vi "RTSequence.Pause.vi"(11 "StimulusProfileReference":refnum<k24>) -> (3 "error out":errorcluster)   [LabVIEW 2013, in "RTSequenceVIs.lvlib"]
uses:
  RTSequenceVIs.lvlib
  NationalInstruments.VeriStand.ClientAPI
  NationalInstruments.VeriStand
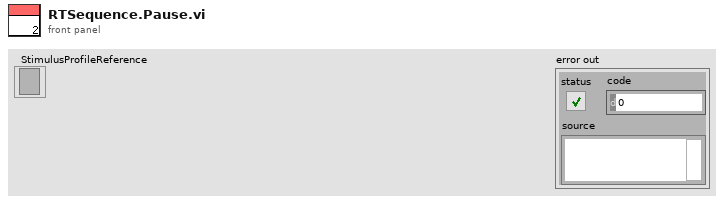
[diagram p1: front panel]
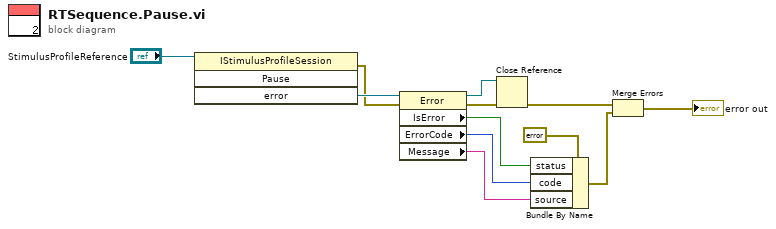
[diagram p0: block diagram]
diagram:
  n1 = invoke class="IStimulusProfileSession" method="Pause"(reference="StimulusProfileReference") -> (error out=w11:errorcluster, "error"=w12:refnum<k24>)  [unwired: 3 in, 2 out]
  n2 = property class="Error"(reference=w12, error in=w11) -> (reference out=w4:refnum<k24>, error out=w5:errorcluster, "IsError"=w6:bool, "ErrorCode"=w7:i32, "Message"=w8:string)
  n3 = Close Reference(reference=w4, error in (no error)=w5) -> (error out=w3:errorcluster)
  n4 = Bundle By Name(cluster=errorcluster {"status"=FALSE, "code"=0, "source"=""} ("error in (no error)"), "status"=w6, "code"=w7, "source"=w8) -> (w2:errorcluster)
  n5 = Merge Errors(w3, w2) -> (→"error out":errorcluster)
